vi "Cannon manual control.vi"() -> ()   [LabVIEW 2012]
panel:
  out "Motor value":dbl
  out "On target":bool
  in  "Throttle value":dbl
  in  "Current angle":dbl
  in  "Min Angle":dbl
  in  "Max Angle":dbl
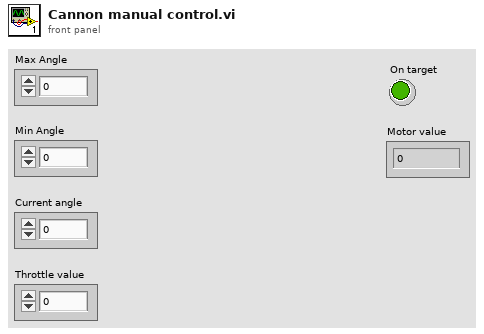
[diagram p1: front panel]
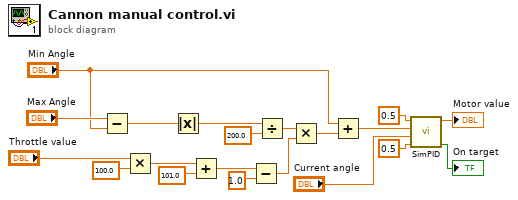
[diagram p0: block diagram]
diagram:
  n1 = Subtract(x="Max Angle", y="Min Angle") -> (x-y=w11:dbl)
  n2 = Multiply(x="Throttle value", y=100.0) -> (x*y=w15:dbl)
  n3 = Absolute Value(x=w11) -> (abs(x)=w3:dbl)
  n4 = Add(x=w15, y=101.0) -> (x+y=w8:dbl)
  n5 = Subtract(x=w8, y=1.0) -> (x-y=w7:dbl)
  n6 = Divide(x=w3, y=200.0) -> (x/y=w1:dbl)
  n7 = Multiply(x=w1, y=w7) -> (x*y=w6:dbl)
  n8 = Add(x="Min Angle", y=w6) -> (x+y=w4:dbl)
  n9 = call "SimPID.vi"("Range"=0.5, "Position"="Current angle", "Set Point"=w4, "Gain"=0.5) -> ("On Target"=→"On target":bool, "result"=→"Motor value":dbl)  [unwired: 5 in]
